vi "Acquisition.vi"(7 "Data Cam Processing en entrée":T1 {"sigma X" format="%0.2f"; "mean X" format="%0.2f"; "mean Y" format="%0.2f"; "sigma Y" format="%0.2f"; "Shutter (us)" scale=22.0..10000000.0; "Gain Caméra" scale=0.0..1023.0}, 8 "entrée d'erreur":errorcluster caption="entrée d'erreur (pas d'erreur)", 10 "Pixel Format":string) -> (0 "sortie d'erreur":errorcluster, 2 "specific error cleared?":bool, 3 "Acquired Frames/s":dbl, 5 "Data Cam Processing en sortie":T1 {"sigma X" format="%0.2f"; "mean X" format="%0.2f"; "mean Y" format="%0.2f"; "sigma Y" format="%0.2f"; "Shutter (us)" scale=22.0..10000000.0; "Gain Caméra" scale=0.0..1023.0})   [LabVIEW 2026]
doc: "Ce vi permet l'acquistion avec la caméra"
uses:
  Data-Processing.ctl
  <vilib>/Serenial/G Industrial Camera/g_industrial_cam/Buffer/Buffer.lvclass
  <vilib>/Serenial/G Industrial Camera/g_industrial_cam/Camera/Camera.lvclass
  <vilib>/picture/picture.llb/imagedata.ctl
  <vilib>/Serenial/G Industrial Camera/g_industrial_cam/Camera/Camera.lvclass/Camera.ctl
  <vilib>/Serenial/G Industrial Camera/g_industrial_cam/Buffer/Buffer.lvclass/Buffer.ctl
  <vilib>/Serenial/G Industrial Camera/g_industrial_cam/Buffer/Read Data as Mono8 Image.vi
  <vilib>/Serenial/G Industrial Camera/g_industrial_cam/Buffer/Access Handle.vi
  <vilib>/Serenial/G Industrial Camera/g_industrial_cam/Camera/Check Not Disconnected.vi
  <vilib>/Serenial/G Industrial Camera/g_industrial_cam/Camera/Check Stream OK.vi
  <vilib>/Utility/error.llb/Error Cluster From Error Code.vi
panel:
  out "Frame Count (inc Errors)":u64
  out "Frame-Error Count":u64
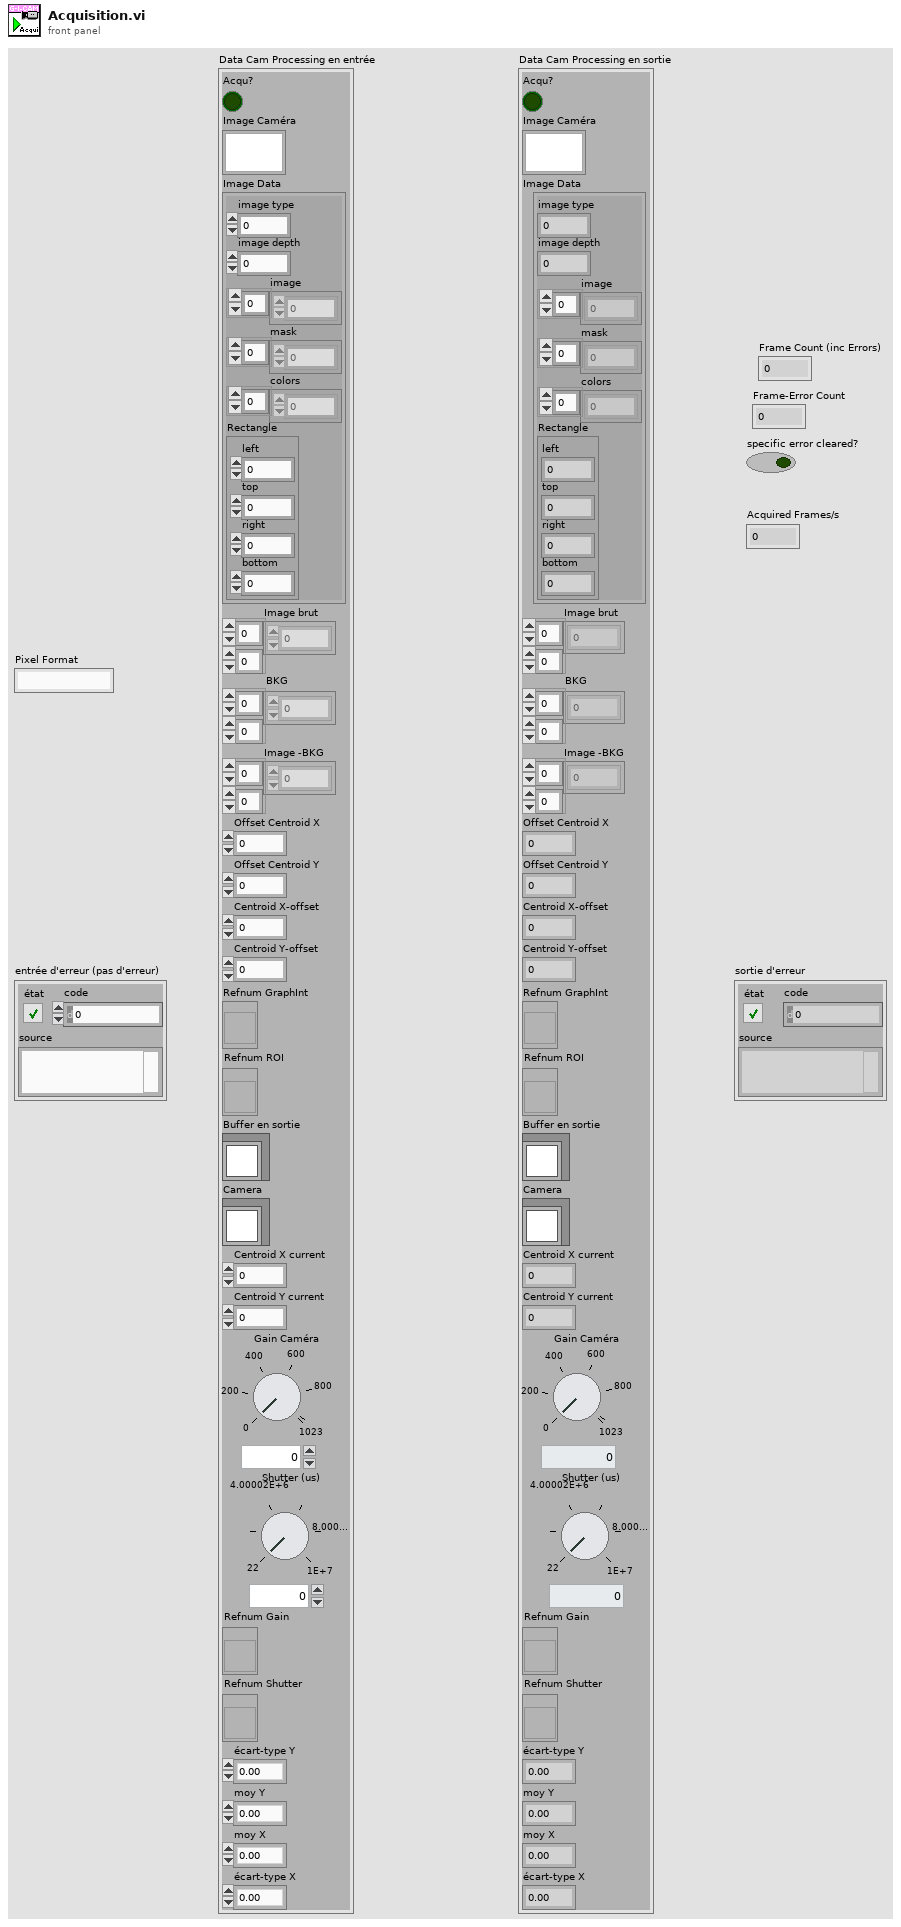
[diagram p1: front panel]
types:
  T1 = typedef "Data-Processing.ctl" = cluster{"Acqu?":bool, "Image Caméra":picture, "Image Data":T2, "Image brut":i16[][], "BKG":i16[][], "Image -BKG":i16[][], "Offset Centroid X":dbl, "Offset Centroid Y":dbl, "Centroid X-offset":dbl, "Centroid Y-offset":dbl, "Refnum GraphInt":refnum<vi>, "Refnum ROI":refnum<vi>, "Buffer en sortie":refnum<class "Buffer.lvclass">, "Camera":refnum<class "Camera.lvclass">, "Centroid X current":dbl, "Centroid Y current":dbl, "Gain Caméra":i32, "Shutter (us)":dbl, "Refnum Gain":refnum<vi>, "Refnum Shutter":refnum<vi>, "sigma Y":dbl, "mean Y":dbl, "mean X":dbl, "sigma X":dbl}
  T2 = typedef "imagedata.ctl" = cluster{"image type":i32, "image depth":i32, "image":u8[], "mask":u8[], "colors":u32[], "Rectangle":cluster{"left":i16, "top":i16, "right":i16, "bottom":i16}}
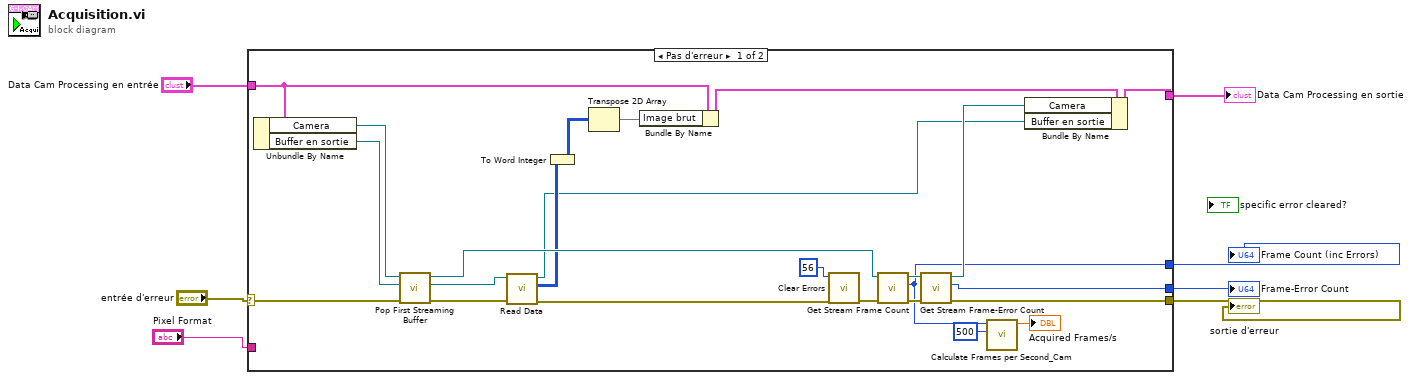
[diagram p0: block diagram]
diagram:
  n1 = case shown="Pas d'erreur" "entrée d'erreur" {
    selector: "entrée d'erreur" -> [w24 w32]
    tunnel: [w15 w33] -> w7
    tunnel: "Data Cam Processing en entrée" -> [w16 w33]
    tunnel: [w30 w32] -> w5
    tunnel: [w29 _] -> w4
    tunnel: [w10 _] -> w3
    tunnel: "Pixel Format" -> [_ _]
    frame No Error {
      n2 = Unbundle By Name(w16) -> ("Camera"=w13:refnum<class "Camera.lvclass">, "Buffer en sortie"=w12:refnum<class "Buffer.lvclass">)
      n3 = call <vilib>:"Pop First Streaming Buffer.vi"("error in (no error)"=w24, "Buffer in"=w12, "Camera in"=w13) -> ("error out"=w22:errorcluster, "Buffer"=w23:refnum<class "Buffer.lvclass">, "Camera"=w31:refnum<class "Camera.lvclass">)  [unwired: 6 in]
      n4 = call-poly <vilib>:"Read Data.vi"("error in (no error)"=w22, "Buffer in"=w23) -> ("error out"=w21:errorcluster, "Image"=w19:u8[][], "Buffer"=w11:refnum<class "Buffer.lvclass">)  [unwired: 7 in]
      n5 = To Word Integer(number=w19) -> (16bit integer=w17:i16[][])
      n6 = Transpose 2D Array(2D array=w17) -> (transposed array=w18:i16[][])
      n7 = Bundle By Name(cluster=w16, "Image brut"=w18) -> (w20:T1)
      n8 = call <vilib>:"Clear Errors.vi"("error in (no error)"=w21, "specific error code to clear (0: all)"=56) -> ("error out"=w25:errorcluster)  [unwired: 4 in, 1 out]
      n9 = call <vilib>:"Get Stream Frame Count.vi"("error in (no error)"=w25, "Camera in"=w31) -> ("error out"=w27:errorcluster, "Frame Count (inc Errors)"=w10:u64, "Camera"=w28:refnum<class "Camera.lvclass">)  [unwired: 7 in]
      n10 = call <vilib>:"Get Stream Frame-Error Count.vi"("error in (no error)"=w27, "Camera in"=w28) -> ("error out"=w30:errorcluster, "Frame-Error Count"=w29:u64, "Camera"=w14:refnum<class "Camera.lvclass">)  [unwired: 7 in]
      n11 = call "Calculate Frames per Second_Cam.vi"("Update Interval (ms)"=u32 500, "Buffer Number"=w10) -> ("Acquired Frames/s"=→"Acquired Frames/s":dbl)  [unwired: 7 in, 2 out]
      n12 = Bundle By Name(cluster=w20, "Camera"=w14, "Buffer en sortie"=w11) -> (w15:T1)
    }
    frame Error {
    }
  }
  "Data Cam Processing en sortie" <- w7
  "sortie d'erreur" <- w5
  "Frame-Error Count" <- w4
  "Frame Count (inc Errors)" <- w3
